vi "PID EGU to Percentage (DBL).vi"(1 "minimum (EGU)":dbl format="%.2f", 2 "input (EGU)":dbl format="%.2f", 3 "maximum (EGU)":dbl format="%.2f") -> (0 "% span":dbl format="%.2f")   [LabVIEW 2020, in "NI_PID_pid.lvlib"]
doc: "Converts an engineering-units input to a percent-of-range output based on the minimum and maximum range settings. Use the DBL instance of this VI to implement a single control loop. Use the DBL Array instance to implement parallel multi-loop control."
uses:
  <vilib>/addons/control/pid/NI_PID_pid.lvlib
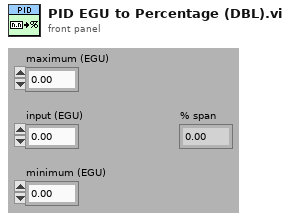
[diagram p1: front panel]
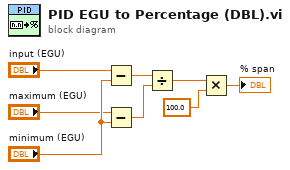
[diagram p0: block diagram]
diagram:
  n1 = Subtract(x="input (EGU)", y="minimum (EGU)") -> (x-y=w5:dbl)
  n2 = Subtract(x="maximum (EGU)", y="minimum (EGU)") -> (x-y=w4:dbl)
  n3 = Divide(x=w5, y=w4) -> (x/y=w2:dbl)
  n4 = Multiply(x=w2, y=100.0) -> (x*y=→"% span":dbl)
